vi "get_slope_from_zero_and_peak.vi"(0 "All in array":cluster{"Array":dbl[], "Amplitudes":dbl[]}[](array[cluster]), 5 "minus-plus crossing?":bool[](array[boolean])) -> (4 "XY Graph":cluster{"Array":dbl[], "Amplitudes":dbl[]}[](graph), 6 "slope":dbl[](array[numeric]), 10 "angle":dbl[](array[numeric]), 12 "slope mean":dbl format="%0.2f", 13 "slope sd":dbl format="%0.2f", 14 "slope variance":dbl format="%0.2f")   [LabVIEW 2020]
uses:
  <vilib>/Analysis/NI_AALBase.lvlib
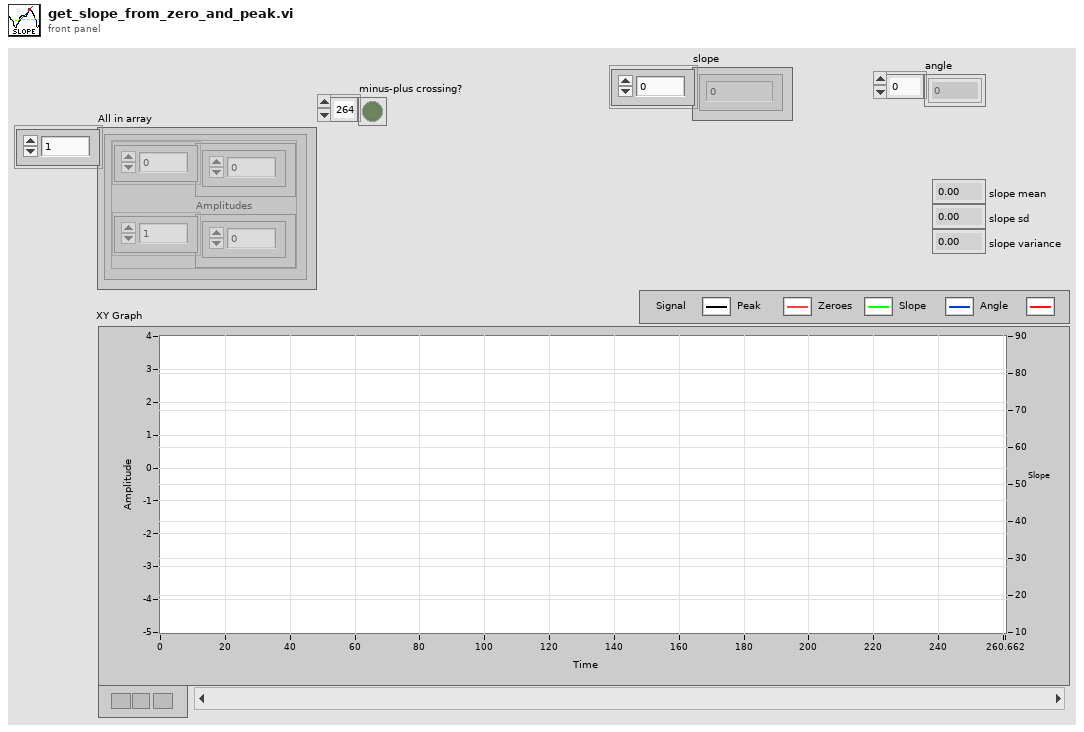
[diagram p1: front panel]
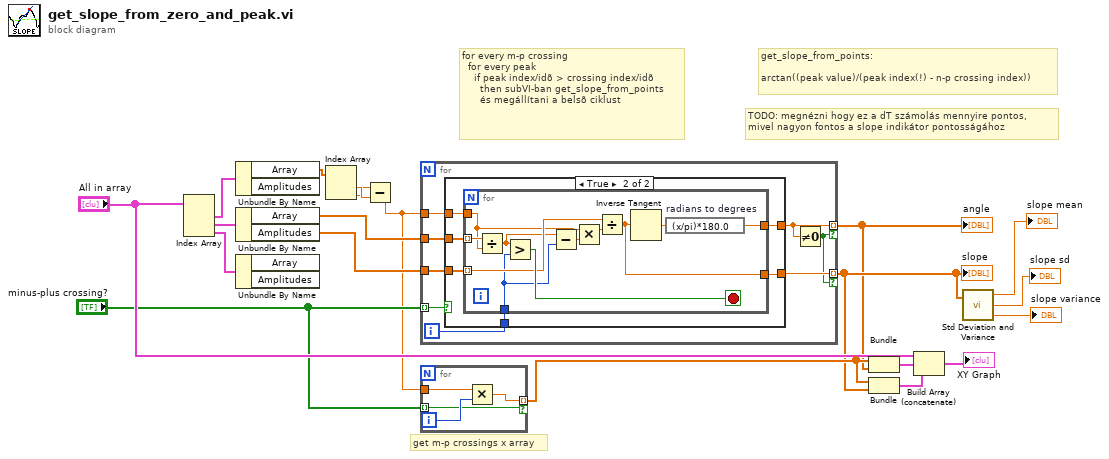
[diagram p0: block diagram]
diagram:
  # "get m-p crossings x array"
  # "TODO: megnézni hogy ez a dT számolás mennyire pontos, \nmivel nagyon fontos a slope indikátor pontosságához"
  # "get_slope_from_points:\n\narctan((peak value)/(peak index(!) - n-p crossing index))"
  # "for every m-p crossing\n  for every peak\n    if peak index/idõ > crossing index/idõ\n      then subVI-ban get_slope_from_points\n      és megállítani a belsõ ciklust"
  n1 = Index Array(array="All in array") -> (element #1=w15:cluster{"Array":dbl[], "Amplitudes":dbl[]}, element #2=w20:cluster{"Array":dbl[], "Amplitudes":dbl[]}, element #3=w19:cluster{"Array":dbl[], "Amplitudes":dbl[]})  [unwired: 3 in]
  n2 = Unbundle By Name(w15) -> ("Array"=w12:dbl[])  [unwired: 1 out]
  n3 = Unbundle By Name(w20) -> ("Array"=w11:dbl[], "Amplitudes"=w16:dbl[])
  n4 = Unbundle By Name(w19) -> ()  [unwired: 2 out]
  n5 = Index Array(array=w12) -> (element #1=w14:dbl, element #2=w13:dbl)  [unwired: 2 in]
  n6 = Subtract(x=w13, y=w14) -> (x-y=w9:dbl)
  n7 = for {
    tunnel: "minus-plus crossing?" -> [w28] mode=indexing
    tunnel: w16 -> [w27]
    tunnel: w9 -> [w26]
    tunnel: w11 -> [w25]
    tunnel: [w23] -> w4 mode=indexing if=w21
    tunnel: [w22] -> w5 mode=indexing if=w21
    i -> [w24]
    n8 = case shown="True" w28 {
      tunnel: w27 -> [_ w34]
      tunnel: w26 -> [_ w33]
      tunnel: w25 -> [_ w32]
      tunnel: w24 -> [_ w31]
      tunnel: [_ w30] -> w23
      tunnel: [_ w29] -> w22
      frame False {
      }
      frame True {
        n9 = for {
          tunnel: w34 -> [w43] mode=indexing
          tunnel: w33 -> [w37]
          tunnel: w32 -> [w45] mode=indexing
          tunnel: w31 -> [w42]
          tunnel: [w39] -> w30
          tunnel: [w35] -> w29
          stop <- w44 stop-if-true
          n10 = Divide(x=w45, y=w37) -> (x/y=w41:dbl)
          n11 = Greater?(x=w41, y=w42) -> (0:w44:bool)
          n12 = Subtract(x=w41, y=w42) -> (x-y=w38:dbl)
          n13 = Multiply(x=w37, y=w38) -> (x*y=w36:dbl)
          n14 = Divide(x=w43, y=w36) -> (x/y=w35:dbl)
          n15 = Inverse Tangent(1:w35) -> (0:w40:dbl)
          n16 = expression code="(x/pi)*180.0" "radians to degrees"(w40) -> (w39:dbl)
        }
      }
    }
    n17 = Not Equal To 0?(x=w23) -> (x != 0?=w21:bool)
  }
  "angle" <- w4
  "slope" <- w5
  n18 = for {
    tunnel: "minus-plus crossing?" -> [w46] mode=indexing
    tunnel: w9 -> [w49]
    tunnel: [w47] -> w6 mode=indexing if=w46
    i -> [w48]
    n19 = Multiply(x=w49, y=w48) -> (x*y=w47:dbl)
  }
  n20 = Bundle(w6, w4) -> (w8:cluster{dbl[], dbl[]})  [unwired: 1 in]
  n21 = Bundle(w6, w5) -> (w7:cluster{dbl[], dbl[]})  [unwired: 1 in]
  n22 = Build Array (concatenate)("All in array", w8, w7) -> (→"XY Graph":cluster{"Array":dbl[], "Amplitudes":dbl[]}[])
  n23 = call <vilib>:"Std Deviation and Variance.vi"("X"=w5) -> ("mean"=→"slope mean":dbl, "standard deviation"=→"slope sd":dbl, "variance"=→"slope variance":dbl)  [unwired: 1 in]
